vi "Start Test.vi"(8 "error in (no error)":errorcluster, 10 "Tests":string[](array[string]), 11 "Coverage Report in":refnum<class "Coverage Report.lvclass">) -> (0 "error out":errorcluster, 3 "Coverage Report out":refnum<class "Coverage Report.lvclass">)   [LabVIEW 2020, in "Coverage Report.lvclass"]
uses:
  Coverage Report.lvclass
  Coverage Report.lvclass/Coverage Report.ctl
  C:/git/astemes-lunit/source/Framework/Report Plugin/Report Plugin.lvclass
  C:/git/astemes-lunit/source/Framework/Plugin/Plugin.lvclass
  C:/git/astemes-lunit/source/Plugins/Coverage Report/Coverage Report.lvclass
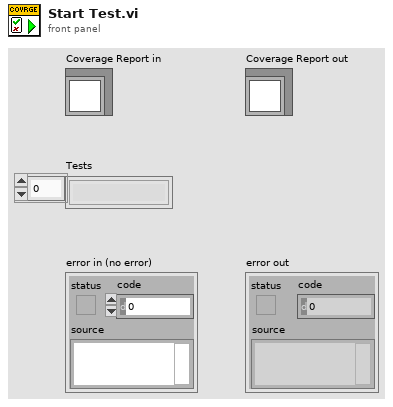
[diagram p1: front panel]
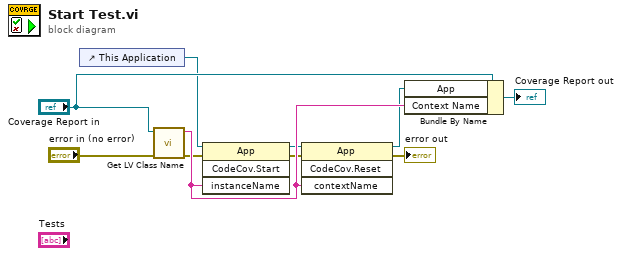
[diagram p0: block diagram]
diagram:
  n1 = control-ref of="This Application"() -> (w1:refnum<vi>)
  n2 = call <vilib>:"Get LV Class Name.vi"("error in (no error)"="error in (no error)", "object"="Coverage Report in") -> ("error out"=w5:errorcluster, "class name"=w6:string)  [unwired: 8 in]
  n3 = invoke class="App" method="CodeCov.Start"(reference=w1, error in=w5, "instanceName"=w6) -> (reference out=w3:refnum<vi>, error out=w2:errorcluster)  [unwired: 1 in, 2 out]
  n4 = invoke class="App" method="CodeCov.Reset"(reference=w3, error in=w2, "contextName"=w6) -> (reference out=w4:refnum<vi>, error out=→"error out":errorcluster)  [unwired: 1 in, 2 out]
  n5 = Bundle By Name(cluster="Coverage Report in", "App"=w4, "Context Name"=w6) -> (→"Coverage Report out":refnum<class "Coverage Report.lvclass">)
